vi "Write Hardware.vi"(8 "error in (no error)":errorcluster, 11 "Sensor & Control in":refnum<class "Control.lvclass">) -> (0 "error out":errorcluster, 3 "Sensor & Control out":refnum<class "Control.lvclass">)   [LabVIEW 2013, in "Control.lvib.lvlib" / "Control.lvclass"]
uses:
  Control.lvclass
  Control.lvclass/Control.ctl
  Read VISA.vi
  PluginInterface/PluginInterface.lvlibp/PluginInterfaceClass/Read DVR.vi
  PluginInterface/PluginInterface.lvlibp/PluginInterfaceClass/Read Name.vi
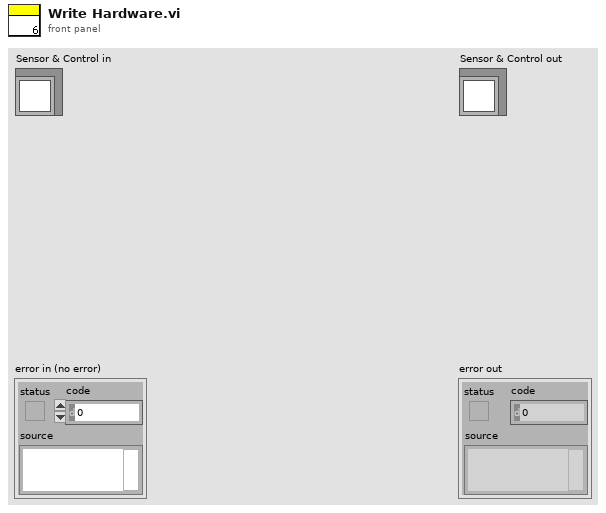
[diagram p1: front panel]
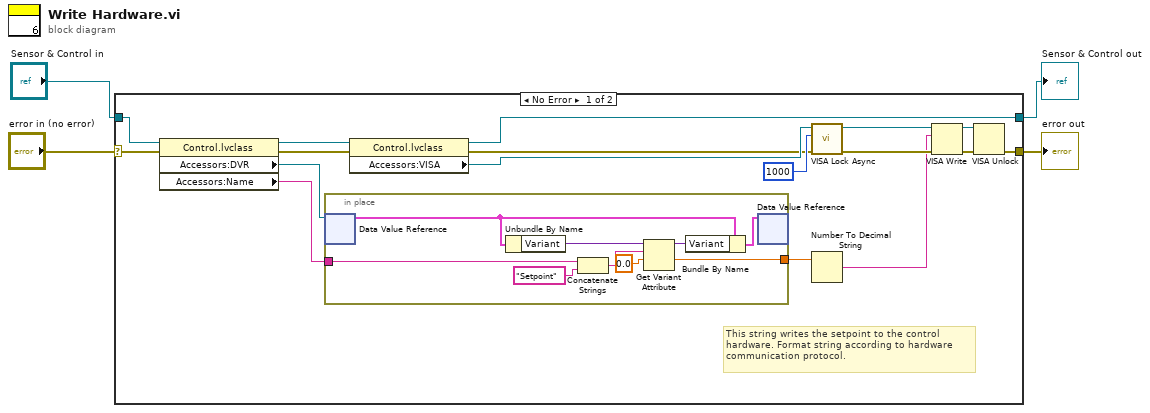
[diagram p0: block diagram]
diagram:
  n1 = case shown="No Error" "error in (no error)" {
    selector: "error in (no error)" -> [w20 w32]
    tunnel: [w8 w32] -> w1
    tunnel: [w17 w31] -> w2
    tunnel: "Sensor & Control in" -> [w21 w31]
    frame No Error {
      # "This string writes the setpoint to the control \nhardware. Format string according to hardware\ncommunication protocol."
      n2 = property class="Control.lvclass"(reference=w21, error in=w20) -> (reference out=w6:refnum<class "Control.lvclass">, error out=w5:errorcluster, "Accessors:DVR"=w19:refnum<data-value>, "Accessors:Name"=w7:string)
      n3 = in-place {
        in-place-border: [w25] -> w16
        in-place-border: w7 -> [w23]
        n4 = in-place-dvr #1(w19) -> (w27:cluster{"Array":string[], "Variant":variant})  [unwired: 1 out]
        n5 = Unbundle By Name(w27) -> ("Variant"=w29:variant)
        n6 = Concatenate Strings(w23, "Setpoint") -> (w22:string)
        n7 = Get Variant Attribute(Variant=w29, name=w22, default value (empty Variant)=0.0) -> (duplicate Variant=w28:variant, value=w25:dbl)  [unwired: 1 in, 2 out]
        n8 = Bundle By Name(cluster=w27, "Variant"=w28) -> (w30:cluster{"Array":string[], "Variant":variant})
        n9 = in-place-dvr #1(w30) -> ()  [unwired: 2 out]
      }
      n10 = property class="Control.lvclass"(reference=w6, error in=w5) -> (reference out=w17:refnum<class "Control.lvclass">, error out=w9:errorcluster, "Accessors:VISA"=w18:refnum<visa-resource-name>)
      n11 = call <vilib>:"VISA Lock Async.vi"("error in (no error)"=w9, "timeout (0)"=u32 1000, "VISA resource name"=w18) -> ("error out"=w14:errorcluster, "VISA resource name out"=w11:refnum<visa-resource-name>)  [unwired: 6 in, 1 out]
      n12 = Number To Decimal String(number=w16) -> (decimal integer string=w10:string)  [unwired: 1 in]
      n13 = VISA Write(VISA resource name=w11, write buffer=w10, error in (no error)=w14) -> (VISA resource name out=w12:refnum<visa-resource-name>, error out=w13:errorcluster)  [unwired: 1 out]
      n14 = VISA Unlock(8:w13, 11:w12) -> (0:w8:errorcluster)  [unwired: 1 out]
    }
    frame Error {
    }
  }
  "error out" <- w1
  "Sensor & Control out" <- w2
